vi "Write Grapes.vi"(8 "error in (no error)":errorcluster, 10 "Grapes":refnum<vi>, 11 "Grape in":refnum<class "Grape.lvclass">) -> (0 "error out":errorcluster, 3 "Grape out":refnum<class "Grape.lvclass">)   [LabVIEW 2021, in "Grape.lvclass"]
uses:
  Grape.lvclass
  Grape.lvclass/Grape.ctl
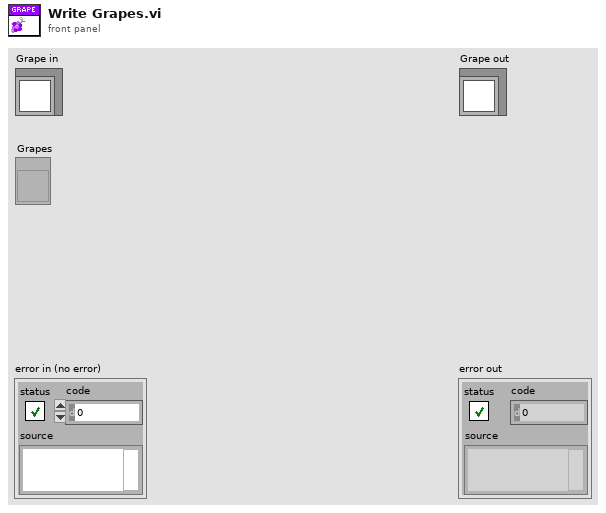
[diagram p1: front panel]
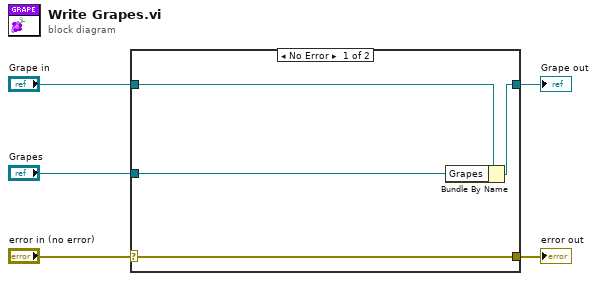
[diagram p0: block diagram]
diagram:
  n1 = case shown="No Error" "error in (no error)" {
    selector: "error in (no error)" -> [w9 w10]
    tunnel: [w9 w10] -> w4
    tunnel: [w7 w11] -> w2
    tunnel: "Grape in" -> [w8 w11]
    tunnel: "Grapes" -> [w6 _]
    frame No Error {
      n2 = Bundle By Name(cluster=w8, "Grapes"=w6) -> (w7:refnum<class "Grape.lvclass">)
    }
    frame Error {
    }
  }
  "error out" <- w4
  "Grape out" <- w2
